vi "Write.vi"(10 "Boolean":bool, 11 "Boolean in":refnum<class "Boolean.lvclass">) -> (3 "Boolean out":refnum<class "Boolean.lvclass">)   [LabVIEW 2020, in "Data.lvlib" / "Boolean.lvclass"]
doc: "Write boolean."
uses:
  Boolean.lvclass
  Boolean.lvclass/Boolean.ctl
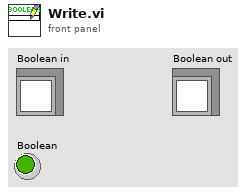
[diagram p1: front panel]
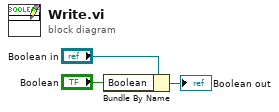
[diagram p0: block diagram]
diagram:
  n1 = Bundle By Name(cluster="Boolean in", "Boolean"="Boolean") -> (→"Boolean out":refnum<class "Boolean.lvclass">)
